vi "execute_value_write_policy.vi"(8 "error in (no error)":errorcluster, 9 "Publish Time":timestamp, 10 "New Topic Value":variant, 11 "WriteWhenVisibleSubscription In":refnum<class "WriteWhenVisibleSubscription.lvclass">) -> (0 "error out":errorcluster, 3 "WriteWhenVisibleSubscription Out":refnum<class "WriteWhenVisibleSubscription.lvclass">)   [LabVIEW 2017, in "SubscriptionPolicy.lvlib" / "WriteWhenVisibleSubscription.lvclass"]
uses:
  WriteWhenVisibleSubscription.lvclass
  C:/Git/mva-framework/Framework/IMediator/ISubscriptionPolicy/ISubscriptionPolicy.lvclass
  WriteWhenVisibleSubscription.lvclass/WriteWhenVisibleSubscription.ctl
  IMediator/ISubscriptionPolicy/ISubscriptionPolicy.lvclass/ISubscriptionPolicy.ctl
  IMediator/ITransport/ITransport.lvclass
  IMediator/ISubscriptionPolicy/ISubscriptionPolicy.lvclass
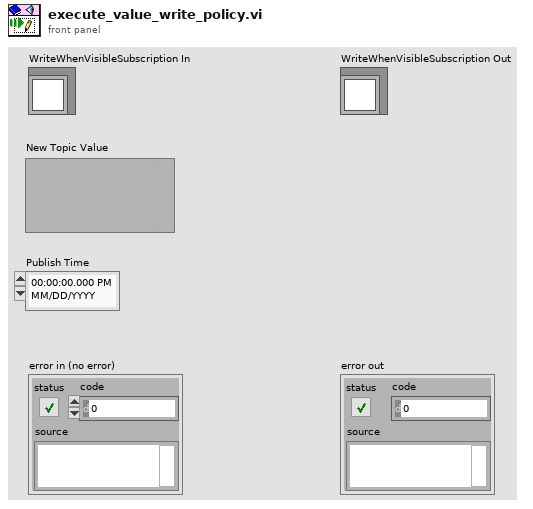
[diagram p1: front panel]
types:
  T1 = enum32{"Invalid", "Standard", "Closed", "Hidden", "Minimized", "Maximized"}
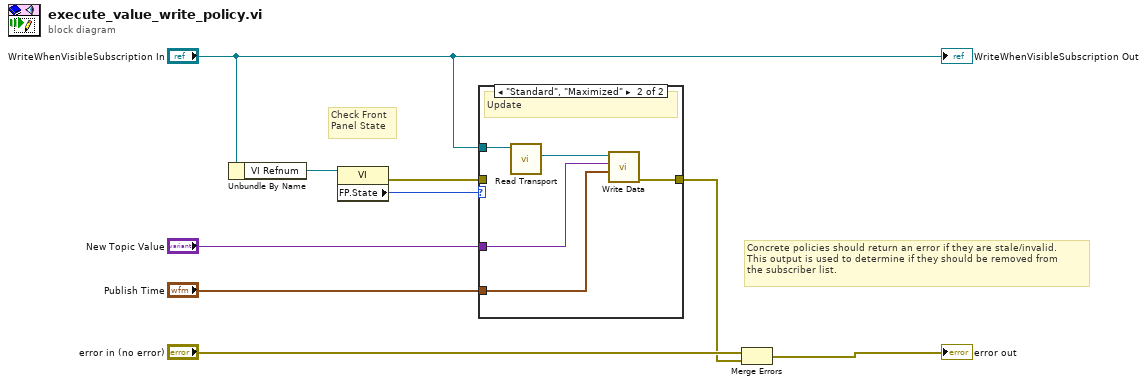
[diagram p0: block diagram]
diagram:
  # "Check Front\nPanel State"
  # "Concrete policies should return an error if they are stale/invalid.\nThis output is used to determine if they should be removed from\nthe subscriber list."
  n1 = Unbundle By Name("WriteWhenVisibleSubscription In") -> ("VI Refnum"=w1:refnum<vi>)
  n2 = property class="VI"(reference=w1) -> (error out=w6:errorcluster, "FP.State"=w7:T1)  [unwired: 1 in, 1 out]
  n3 = case shown="\"Standard\", \"Maximized\"" w7 {
    tunnel: "New Topic Value" -> [_ w15]
    tunnel: "Publish Time" -> [_ w14]
    tunnel: [w10 w13] -> w3
    tunnel: "WriteWhenVisibleSubscription In" -> [_ w11]
    tunnel: w6 -> [w10 _]
    frame Default {
      # "No update"
    }
    frame "Standard", "Maximized" {
      # "Update"
      n4 = call "Read Transport.vi"("ISubscriptionPolicy in"=w11) -> ("Transport"=w12:refnum<class "ITransport.lvclass">)  [unwired: 10 in]
      n5 = call-dynamic "Write Data.vi"("Publication Time"=w14, "Value"=w15, "ITransport in"=w12) -> ("error out"=w13:errorcluster)  [unwired: 7 in, 1 out]
    }
  }
  n6 = Merge Errors("error in (no error)", w3) -> (→"error out":errorcluster)
  "WriteWhenVisibleSubscription Out" <- "WriteWhenVisibleSubscription In"
